vi "Post_Build_RemoveExtraFiles.vi"(8 "error in (no error)":errorcluster, 10 "Rumtime Name":string, 11 "Files to remove":path[](array[path])) -> (0 "error out":errorcluster)   [LabVIEW 2017]
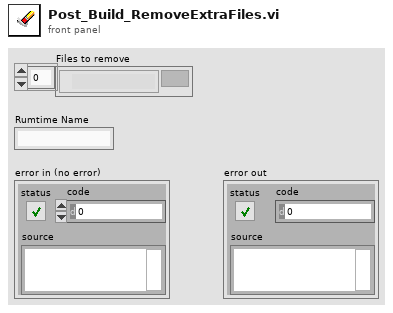
[diagram p1: front panel]
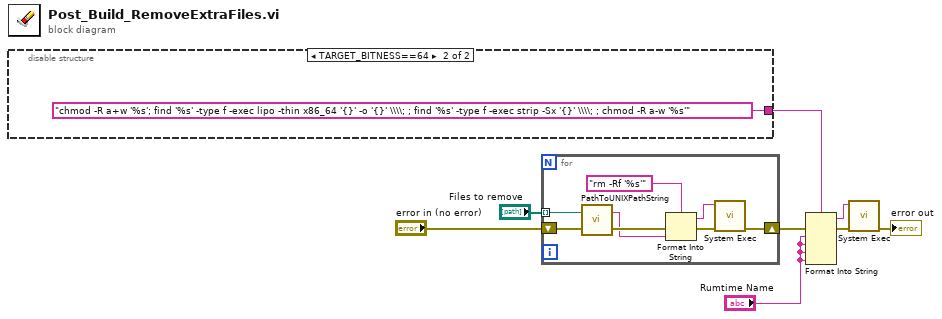
[diagram p0: block diagram]
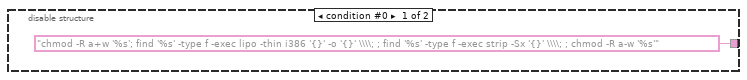
[diagram p2: hidden frame]
diagram:
  n1 = disable-structure shown="TARGET_BITNESS==64" {
    disable-tunnel: ["chmod -R a+w '%s'; find '%s' -type f -exec lipo -thin i386 '{}' -o '{}' \\\\; ; find '%s' -type f -exec strip -Sx '{}' \\\\; ; chmod -R a-w '%s'" ("format string") "chmod -R a+w '%s'; find '%s' -type f -exec lipo -thin x86_64 '{}' -o '{}' \\\\; ; find '%s' -type f -exec strip -Sx '{}' \\\\; ; chmod -R a-w '%s'" ("format string")] -> w8
    frame condition #0 {
    }
    frame condition #1 (active) {
    }
  }
  n2 = for {
    tunnel: "Files to remove" -> [w18] mode=indexing
    shift-right: [w14] -> w5
    shift-left: "error in (no error)" -> [w17]
    n3 = call <vilib>:"PathToUNIXPathString.vi"("error in (no error)"=w17, "LV Path"=w18) -> ("error out"=w16:errorcluster, "UNIX Path"=w12:string)
    n4 = Format Into String(format string="rm -Rf '%s'", error in=w16, w12) -> (resulting string=w13:string, error out=w15:errorcluster)  [unwired: 1 in]
    n5 = call <vilib>:"System Exec.vi"("error in (no error)"=w15, "command line"=w13) -> ("error out"=w14:errorcluster)  [unwired: 6 in, 3 out]
  }
  n6 = Format Into String(format string=w8, error in=w5, "Rumtime Name", "Rumtime Name", "Rumtime Name", "Rumtime Name") -> (resulting string=w4:string, error out=w3:errorcluster)  [unwired: 1 in]
  n7 = call <vilib>:"System Exec.vi"("error in (no error)"=w3, "command line"=w4) -> ("error out"=→"error out":errorcluster)  [unwired: 6 in, 3 out]
